vi "Git_CheckUpdate.vi"(4 "Your Password (not necessary)":string, 5 "Current Version Date (YYYY-MM-DD)":string, 6 "Your User Name (not necessary)":string, 7 "Current Version Number (vX.XX)":string, 8 "error in":errorcluster, 10 "Repo Name":string, 11 "Repo User Name":string) -> (0 "error out":errorcluster, 2 "Zip Address":string, 3 "Update?":bool)   [LabVIEW 2012]
doc: "Checks whether the specified username/repo is up to date compared to the input version number and date."
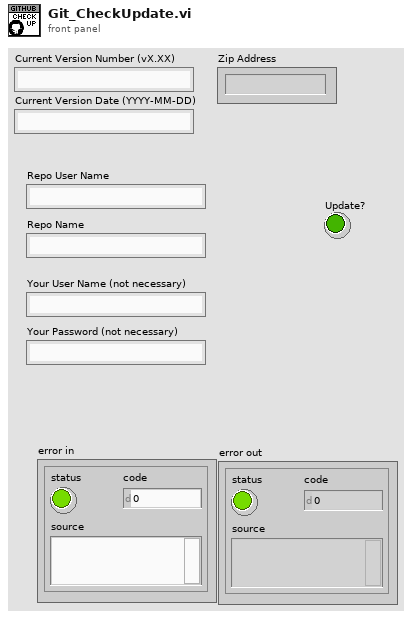
[diagram p1: front panel]
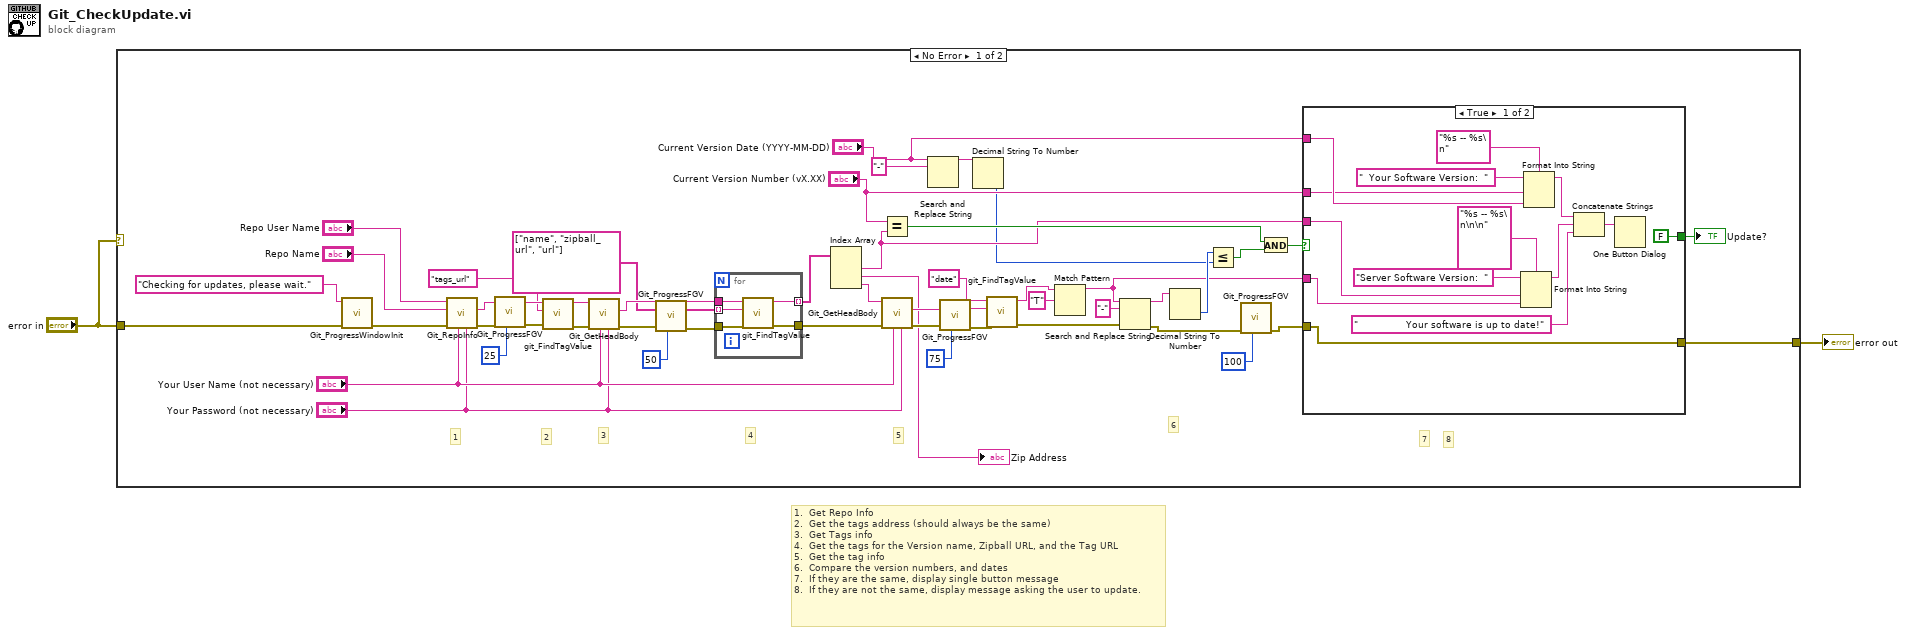
[diagram p0: block diagram]
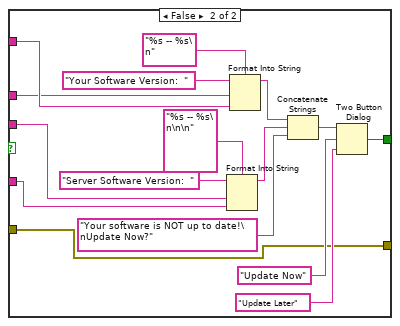
[diagram p2: hidden frame]
diagram:
  # "1.  Get Repo Info\n2.  Get the tags address (should always be the same)\n3.  Get Tags info\n4.  Get the tags for the Version name, Zipball URL, and the Tag URL\n5.  Get the tag info\n6.  Compare the version numbers, and dates\n7.  If they are the same, display single button message\n8.  If they are not the same, display message asking the user to update."
  n1 = case shown="No Error" "error in" {
    tunnel: "error in" -> [w20 w87]
    tunnel: [w21 w87] -> w2
    frame No Error {
      # "8"
      # "7"
      # "6"
      # "5"
      # "4"
      # "3"
      # "2"
      # "1"
      n2 = call "Git_ProgressWindowInit.vi"("error in (no error)"=w20, "Message"="Checking for updates, please wait.") -> ("error out"=w19:errorcluster)  [unwired: 7 in, 2 out]
      n3 = call "Git_RepoInfo.vi"("Your Password (not necessary)"="Your Password (not necessary)", "Your User Name (not necessary)"="Your User Name (not necessary)", "error in (no error)"=w19, "Repo Name"="Repo Name", "Repo User Name"="Repo User Name") -> ("error out"=w18:errorcluster, "body"=w49:string)  [unwired: 3 in, 2 out]
      n4 = call "Git_ProgressFGV.vi"("Update"=u8 25 ("Slide"), "Error In"=w18) -> ("Error Out"=w17:errorcluster)  [unwired: 9 in]
      n5 = call "git_FindTagValue.vi"("Error In"=w17, "Tag Name"="tags_url", "Text"=w49) -> ("Error Out"=w47:errorcluster, "Value"=w46:string)  [unwired: 4 in, 3 out]
      n6 = call "Git_GetHeadBody.vi"("Your Password (not necessary)"="Your Password (not necessary)", "Your User Name (not necessary)"="Your User Name (not necessary)", "error in (no error)"=w47, "Address"=w46) -> ("error out"=w13:errorcluster, "body"=w45:string)  [unwired: 5 in, 1 out]
      n7 = call "Git_ProgressFGV.vi"("Update"=u8 50 ("Slide"), "Error In"=w13) -> ("Error Out"=w14:errorcluster)  [unwired: 9 in]
      n8 = for {
        tunnel: w14 -> [w86]
        tunnel: w45 -> [w85]
        tunnel: string[] ["name", "zipball_url", "url"] -> [w84] mode=indexing
        tunnel: [w83] -> w6
        tunnel: [w82] -> w43 mode=indexing
        n9 = call "git_FindTagValue.vi"("Error In"=w86, "Tag Name"=w84, "Text"=w85) -> ("Error Out"=w83:errorcluster, "Value"=w82:string)  [unwired: 4 in, 3 out]
      }
      n10 = Index Array(array=w43) -> (element #1=w25:string, element #2=→"Zip Address":string, element #3=w42:string)  [unwired: 3 in]
      n11 = Equal?(x="Current Version Number (vX.XX)", y=w25) -> (x = y?=w29:bool)
      n12 = call "Git_GetHeadBody.vi"("Your Password (not necessary)"="Your Password (not necessary)", "Your User Name (not necessary)"="Your User Name (not necessary)", "error in (no error)"=w6, "Address"=w42) -> ("error out"=w5:errorcluster, "body"=w39:string)  [unwired: 5 in, 1 out]
      n13 = Search and Replace String(input string="Current Version Date (YYYY-MM-DD)", search string="-") -> (result string=w33:string)  [unwired: 6 in, 3 out]
      n14 = call "Git_ProgressFGV.vi"("Update"=u8 75 ("Slide"), "Error In"=w5) -> ("Error Out"=w4:errorcluster)  [unwired: 9 in]
      n15 = Decimal String To Number(string=w33) -> (number=w7:i32)  [unwired: 2 in, 1 out]
      n16 = call "git_FindTagValue.vi"("Error In"=w4, "Tag Name"="date", "Text"=w39) -> ("Error Out"=w27:errorcluster, "Value"=w37:string)  [unwired: 4 in, 3 out]
      n17 = Match Pattern(string=w37, regular expression="T") -> (before substring=w23:string)  [unwired: 1 in, 3 out]
      n18 = Search and Replace String(input string=w23, search string="-", error in=w27) -> (result string=w32:string, error out=w10:errorcluster)  [unwired: 5 in, 2 out]
      n19 = Decimal String To Number(string=w32) -> (number=w31:i32)  [unwired: 2 in, 1 out]
      n20 = Less Or Equal?(x=w31, y=w7) -> (x <= y?=w30:bool)
      n21 = call "Git_ProgressFGV.vi"("Update"=u8 100 ("Slide"), "Error In"=w10) -> ("Error Out"=w9:errorcluster)  [unwired: 9 in]
      n22 = And(x=w29, y=w30) -> (x .and. y?=w28:bool)
      n23 = case shown="True" w28 {
        tunnel: w9 -> [w52 w66]
        tunnel: "Current Version Number (vX.XX)" -> [w64 w80]
        tunnel: w25 -> [w59 w75]
        tunnel: "Current Version Date (YYYY-MM-DD)" -> [w65 w81]
        tunnel: w23 -> [w58 w74]
        tunnel: [FALSE ("T button?") w67] -> w22
        tunnel: [w52 w66] -> w21
        frame True {
          n24 = Format Into String(format string="%s -- %s\n\n\n", initial string="Server Software Version:  ", w59, w58) -> (resulting string=w56:string)  [unwired: 1 in, 1 out]
          n25 = Format Into String(format string="%s -- %s\n", initial string="  Your Software Version:  ", w64, w65) -> (resulting string=w57:string)  [unwired: 1 in, 1 out]
          n26 = Concatenate Strings(w57, w56, "                Your software is up to date!" ("message")) -> (w54:string)
          n27 = One Button Dialog(message=w54) -> ()  [unwired: 1 in, 1 out]
        }
        frame False {
          n28 = Format Into String(format string="%s -- %s\n\n\n", initial string="Server Software Version:  ", w75, w74) -> (resulting string=w72:string)  [unwired: 1 in, 1 out]
          n29 = Format Into String(format string="%s -- %s\n", initial string="Your Software Version:  ", w80, w81) -> (resulting string=w73:string)  [unwired: 1 in, 1 out]
          n30 = Concatenate Strings(w73, w72, "Your software is NOT up to date!\nUpdate Now?" ("message")) -> (w70:string)
          n31 = Two Button Dialog(message=w70, 1:"Update Later" ("T button name (\"OK\")"), 2:"Update Now" ("T button name (\"OK\")")) -> (T button?=w67:bool)
        }
      }
      "Update?" <- w22
    }
    frame Error {
    }
  }
  "error out" <- w2
